vi "仪器日志.vi"(11 "质控仪器状态显示":T1) -> (3 "仪器日志":string)   [LabVIEW 2016, in "质控单元V2.lvlib"]
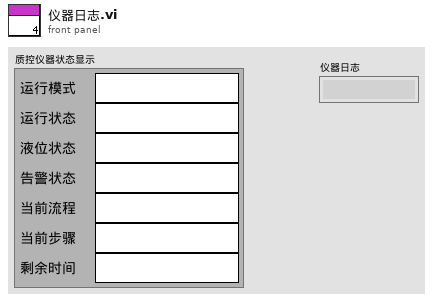
[diagram p1: front panel]
types:
  T1 = typedef "质控单元V2.lvlib/质控仪器状态显示.ctl" = cluster{"运行模式":string, "运行状态":string, "液位状态":string, "告警状态":string, "当前流程":string, "当前步骤":string, "剩余时间":string}
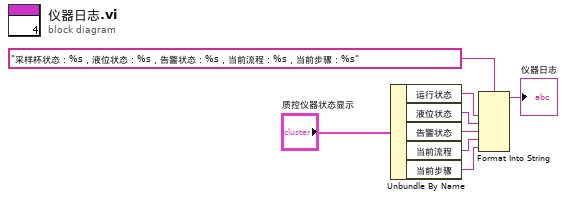
[diagram p0: block diagram]
diagram:
  n1 = Unbundle By Name("质控仪器状态显示") -> ("运行状态"=w3:string, "液位状态"=w4:string, "告警状态"=w5:string, "当前流程"=w6:string, "当前步骤"=w7:string)
  n2 = Format Into String(format string="采样杯状态：%s，液位状态：%s，告警状态：%s，当前流程：%s，当前步骤：%s" ("格式字符串"), w3, w4, w5, w6, w7) -> (resulting string=→"仪器日志":string)  [unwired: 2 in, 1 out]
